vi "Write Drive Train Status Ref.vi"(8 "error in (no error)":errorcluster, 10 "Drive Train Status Ref":refnum<vi>, 11 "Drive Train in":refnum<class "Drive Train.lvclass">) -> (0 "error out":errorcluster, 3 "Drive Train out":refnum<class "Drive Train.lvclass">)   [LabVIEW 2014, in "Logical Systems.lvlib" / "Drive Train.lvlib" / "Drive Train.lvclass"]
uses:
  Drive Train.lvclass
  Drive Train Status.ctl
  Drive Train.lvclass/Drive Train.ctl
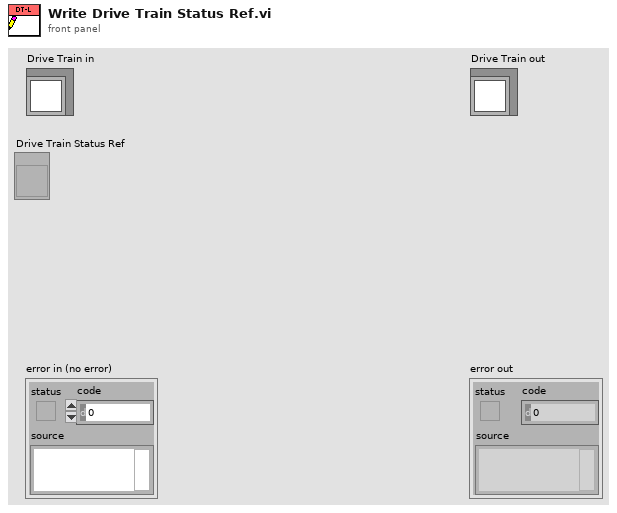
[diagram p1: front panel]
types:
  T1 = typedef "Logical Systems.lvlib/Drive Train.lvlib/Drive Train.lvclass/Drive Train Status.ctl" = cluster{"Left Power":dbl, "Right Power":dbl, "Left Power Setpoint":dbl, "Right Power Setpoint":dbl}
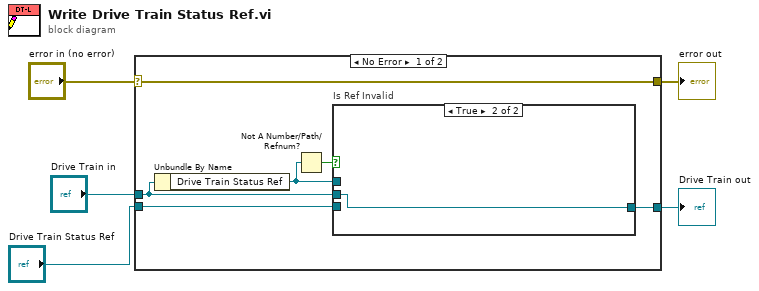
[diagram p0: block diagram]
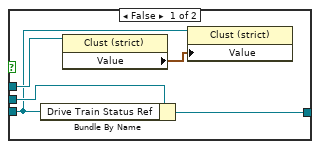
[diagram p2: hidden frame]
diagram:
  n1 = case shown="No Error" "error in (no error)" {
    selector: "error in (no error)" -> [w11 w18]
    tunnel: [w11 w18] -> w4
    tunnel: [w10 w19] -> w2
    tunnel: "Drive Train in" -> [w8 w19]
    tunnel: "Drive Train Status Ref" -> [w9 _]
    frame No Error {
      n2 = Unbundle By Name(w8) -> ("Drive Train Status Ref"=w6:refnum<vi>)
      n3 = Not A Number/Path/Refnum?(number/path/refnum=w6) -> (NaN/Path/Refnum?=w7:bool)
      n4 = case "Is Ref Invalid" shown="True" w7 {
        tunnel: [w16 w17] -> w10
        tunnel: w9 -> [w13 _]
        tunnel: w8 -> [w15 w17]
        tunnel: w6 -> [w14 _]
        frame False {
          n5 = Bundle By Name(cluster=w15, "Drive Train Status Ref"=w13) -> (w16:refnum<class "Drive Train.lvclass">)
          n6 = property class="Clust (strict)"(reference=w14) -> ("Value"=w12:T1)  [unwired: 1 in, 2 out]
          n7 = property class="Clust (strict)"(reference=w13, "Value"=w12) -> ()  [unwired: 1 in, 2 out]
        }
        frame True {
        }
      }
    }
    frame Error {
    }
  }
  "error out" <- w4
  "Drive Train out" <- w2
